vi "CTRE_Phoenix_CANcoder_GetStickyFaults.vi"(8 "error in":errorcluster, 11 "CTRE_CANcoder_DeviceRef":T1) -> (0 "error out":errorcluster, 2 "Sticky Faults":T2, 3 "CTRE_CANcoder_DeviceRef":T1)   [LabVIEW 2019]
doc: "Gets the current sticky fault status of the CANcoder."
uses:
  <vilib>/Rock Robotics/WPI/ThirdParty/Phoenix-LabVIEW/CANCoder/Controls/CTRE_Phoenix_CANcoder_DeviceRef.ctl
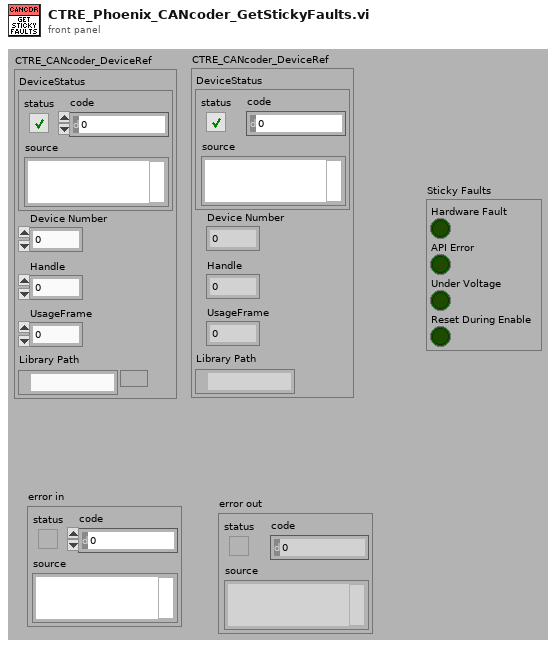
[diagram p1: front panel]
types:
  T1 = typedef "CTRE_Phoenix_CANcoder_DeviceRef.ctl" = cluster{"DeviceStatus":errorcluster, "Device Number":u8, "Handle":u64, "UsageFrame":u32, "Library Path":path}
  T2 = cluster{"Hardware Fault":bool, "API Error":bool, "Under Voltage":bool, "Reset During Enable":bool}
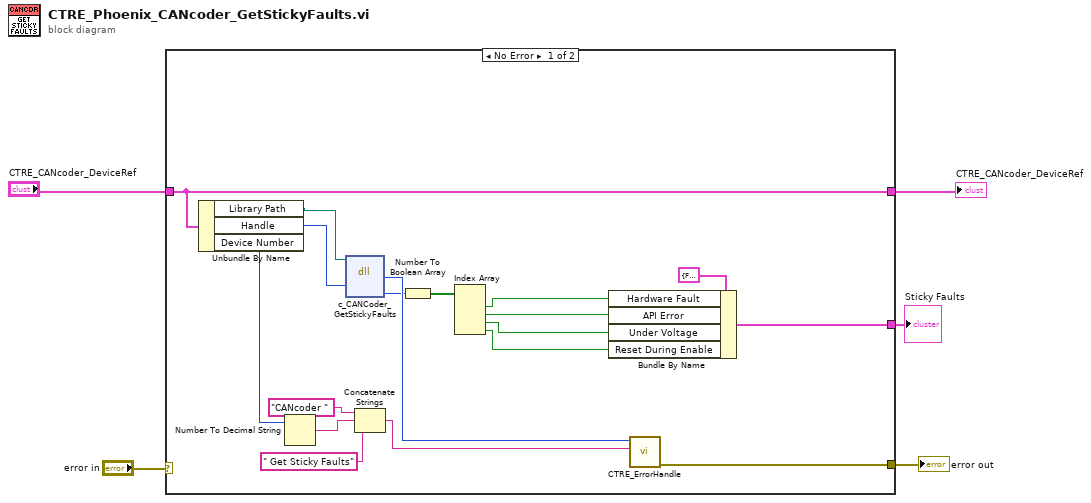
[diagram p0: block diagram]
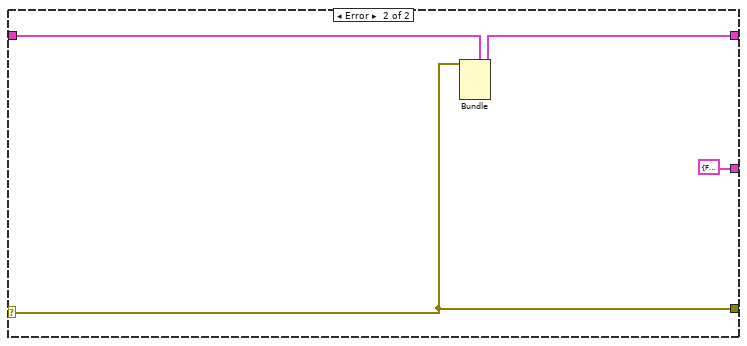
[diagram p2: hidden frame]
diagram:
  n1 = case shown="No Error" "error in" {
    selector: "error in" -> [_ w26]
    tunnel: "CTRE_CANcoder_DeviceRef" -> [w11 w27]
    tunnel: [w23 w26] -> w5
    tunnel: [w11 w25] -> w1
    tunnel: [w14 T2 {"Hardware Fault"=FALSE, "API Error"=FALSE, "Under Voltage"=FALSE, "Reset During Enable"=FALSE} ("Cluster")] -> w3
    frame No Error {
      n2 = Unbundle By Name(w11) -> ("Library Path"=w10:path, "Handle"=w9:u64, "Device Number"=w8:u8)
      n3 = Number To Decimal String(number=w8) -> (decimal integer string=w13:string)  [unwired: 1 in]
      n4 = dll-call lib="?" fn="c_CANCoder_GetStickyFaults"(path in=w10, "handle"=w9) -> ("ErrorCode"=w22:i32, "faults"=w21:i32)  [unwired: 4 in, 2 out]
      n5 = Concatenate Strings("CANcoder " ("string"), w13, " Get Sticky Faults" ("string")) -> (w7:string)
      n6 = Number To Boolean Array(number=w21) -> (Boolean array=w20:bool[])
      n7 = Index Array(array=w20) -> (element #1=w18:bool, element #2=w17:bool, element #3=w16:bool, element #4=w15:bool)  [unwired: 4 in]
      n8 = Bundle By Name(cluster=T2 {"Hardware Fault"=FALSE, "API Error"=FALSE, "Under Voltage"=FALSE, "Reset During Enable"=FALSE}, "Hardware Fault"=w18, "API Error"=w17, "Under Voltage"=w16, "Reset During Enable"=w15) -> (w14:T2)
      n9 = call <vilib>:"CTRE_ErrorHandle.vi"("origin"=w7, "code"=w22) -> ("error out"=w23:errorcluster)  [unwired: 9 in]
    }
    frame Error {
      n10 = Bundle(cluster=w27, "DeviceStatus"=w26) -> (w25:T1)  [unwired: 4 in]
    }
  }
  "error out" <- w5
  "Sticky Faults" <- w3
  "CTRE_CANcoder_DeviceRef" <- w1
